vi "ao-amp_test.vi"() -> ()   [LabVIEW 2020]
uses:
  <instrlib>/niDMM/nidmm.llb/niDMM Function.ctl
  <instrlib>/niDMM/nidmm.llb/niDMM Resolution in Digits.ctl
  <instrlib>/niDMM/nidmm.llb/niDMM Configure Measurement Digits.vi
panel:
  in  "Relay 2":refnum<visa-resource-name>="PXI3::9::INSTR"
  in  "Matrix 3":refnum<visa-resource-name>="PXI14::13::INSTR"
  in  "Matrix 2":refnum<visa-resource-name>="PXI14::13::INSTR"
  in  "Resolution in Digits":T1=5.5 items=["3 1/2"=3.5, "4 1/2"=4.5, "5 1/2"=5.5, "6 1/2"=6.5, "7 1/2"=7.5]
  in  "Measurement Type":T2
  out "Signal Out of Range":bool
  in  "Device Name":refnum<k15>="Multimeter"
  in  "Range (Volts)":dbl=10.0 format="%.2p"
  out "Measurement (Volts)":dbl format="%_7p"
  out "error out":errorcluster
  in  "Relay":refnum<visa-resource-name>="PXI3::9::INSTR"
  in  "Matrix":refnum<visa-resource-name>="PXI14::13::INSTR"
  in  "Gain (x1)":u32(ring)=1 items=["x1"=1, "x2"=2, "x5"=3, "x7"=4, "x10"=5, "x14"=6, "x20"=7]
  in  "Channel (CH1)":u32(ring)=1 items=["CH1"=1, "CH2"=2, "CH3"=3, "CH4"=4, "CH5"=5]
  in  "amplifier":refnum<visa-resource-name>="PXI23::10::INSTR" caption="resource name"
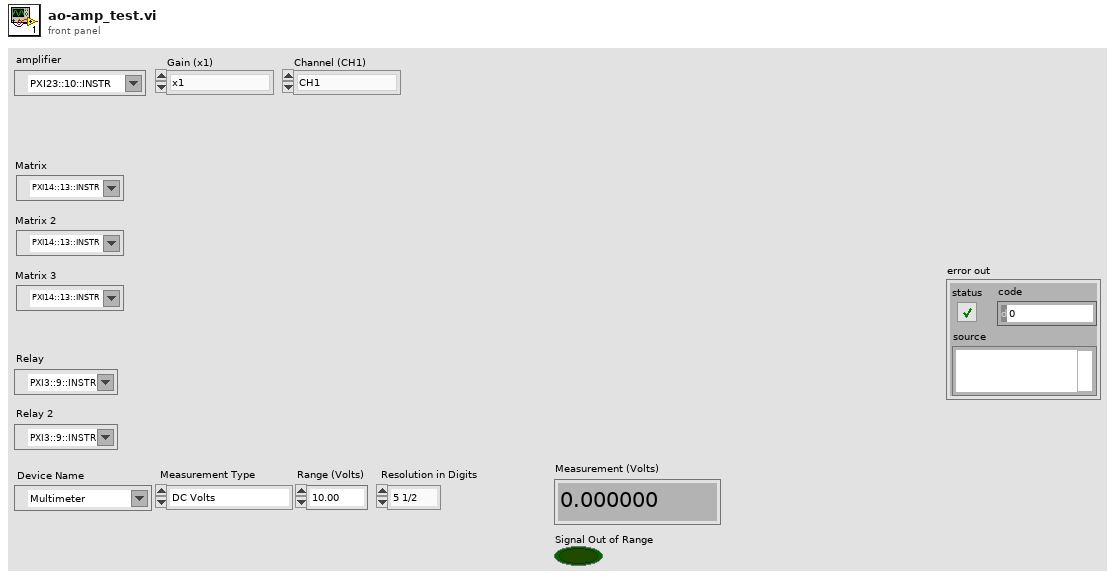
[diagram p1: front panel]
types:
  T1 = typedef "niDMM Resolution in Digits.ctl" = dbl
  T2 = typedef "niDMM Function.ctl" = enum16{"DC Volts", "AC Volts", "DC Current", "AC Current", "2-wire Resistance", "4-wire Resistance", "Diode", "Frequency", "Period", "AC Volts DC Coupled", "Capacitance", "Inductance", "Temperature"}
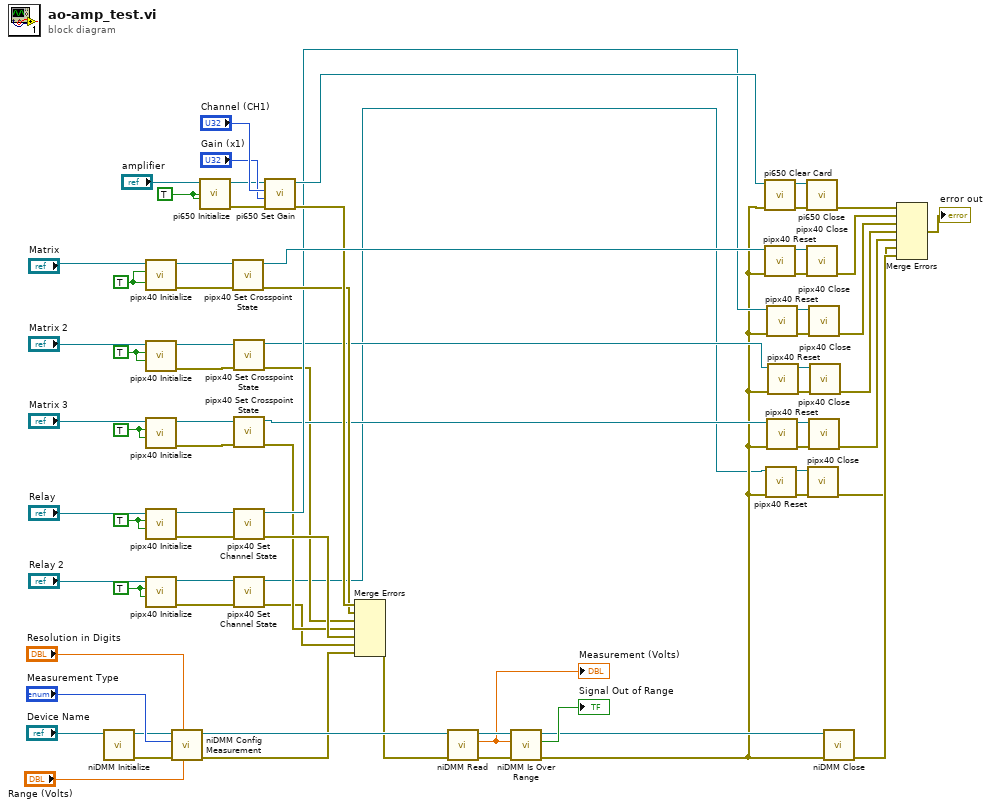
[diagram p0: block diagram]
diagram:
  w14 = TRUE ("id query")
  w25 = TRUE ("id query")
  w26 = TRUE ("id query")
  w50 = TRUE ("id query")
  w63 = TRUE
  w72 = TRUE ("id query (Do Query)")
  n1 = call <instrlib>:"niDMM Initialize.vi"("Instrument Descriptor"="Device Name") -> ("error out"=w33:errorcluster, "instrument handle out"=w32:refnum<k15>)  [unwired: 9 in]
  n2 = call <instrlib>:"pipx40 Initialize.vi"("reset device"=w63, "id query"=w63, "resource name"="Matrix") -> ("error out"=w60:errorcluster, "instrument handle out"=w59:refnum<visa-resource-name>)  [unwired: 7 in]
  n3 = call <instrlib>:"pipx40 Initialize.vi"("reset device"=w26, "id query"=w26, "resource name"="Matrix 2") -> ("error out"=w30:errorcluster, "instrument handle out"=w28:refnum<visa-resource-name>)  [unwired: 7 in]
  n4 = call <instrlib>:"pipx40 Initialize.vi"("reset device"=w25, "id query"=w25, "resource name"="Matrix 3") -> ("error out"=w29:errorcluster, "instrument handle out"=w27:refnum<visa-resource-name>)  [unwired: 7 in]
  n5 = call <instrlib>:"pipx40 Initialize.vi"("reset device"=w50, "id query"=w50, "resource name"="Relay") -> ("error out"=w51:errorcluster, "instrument handle out"=w52:refnum<visa-resource-name>)  [unwired: 7 in]
  n6 = call <instrlib>:"pipx40 Initialize.vi"("reset device"=w14, "id query"=w14, "resource name"="Relay 2") -> ("error out"=w13:errorcluster, "instrument handle out"=w12:refnum<visa-resource-name>)  [unwired: 7 in]
  n7 = call-poly <instrlib>:"niDMM Config Measurement.vi"("Range"="Range (Volts)", "Resolution in Digits"="Resolution in Digits", "error in (no error)"=w33, "Function"="Measurement Type", "instrument handle"=w32) -> ("error out"=w8:errorcluster, "instrument handle out"=w40:refnum<k15>)  [unwired: 5 in]
  n8 = call <instrlib>:"pi650 Initialize.vi"("reset device (Reset Device)"=w72, "id query (Do Query)"=w72, "resource name"="amplifier") -> ("error out"=w66:errorcluster, "instrument handle out"=w67:refnum<visa-resource-name>)  [unwired: 7 in]
  n9 = call <instrlib>:"pipx40 Set Crosspoint State.vi"("error in (no error)"=w60, "instrument handle"=w59) -> ("error out"=w56:errorcluster, "instrument handle out"=w58:refnum<visa-resource-name>)  [unwired: 8 in]
  n10 = call <instrlib>:"pipx40 Set Crosspoint State.vi"("error in (no error)"=w30, "instrument handle"=w28) -> ("error out"=w10:errorcluster, "instrument handle out"=w16:refnum<visa-resource-name>)  [unwired: 8 in]
  n11 = call <instrlib>:"pipx40 Set Crosspoint State.vi"("error in (no error)"=w29, "instrument handle"=w27) -> ("error out"=w9:errorcluster, "instrument handle out"=w15:refnum<visa-resource-name>)  [unwired: 8 in]
  n12 = call <instrlib>:"pipx40 Set Channel State.vi"("error in (no error)"=w51, "instrument handle"=w52) -> ("error out"=w49:errorcluster, "instrument handle out"=w45:refnum<visa-resource-name>)  [unwired: 8 in]
  n13 = call <instrlib>:"pipx40 Set Channel State.vi"("error in (no error)"=w13, "instrument handle"=w12) -> ("error out"=w7:errorcluster, "instrument handle out"=w1:refnum<visa-resource-name>)  [unwired: 8 in]
  n14 = call <instrlib>:"pi650 Set Gain.vi"("error in (no error)"=w66, "Gain (x1)"="Gain (x1)", "Channel (CH1)"="Channel (CH1)", "instrument handle"=w67) -> ("error out"=w57:errorcluster, "instrument handle out"=w65:refnum<visa-resource-name>)  [unwired: 6 in]
  n15 = Merge Errors(w57, w56, w10, w9, w49, w7, w8) -> (w31:errorcluster)
  n16 = call <instrlib>:"niDMM Read.vi"("error in (no error)"=w31, "instrument handle"=w40) -> ("error out"=w39:errorcluster, "Measurement"=w37:dbl, "instrument handle out"=w38:refnum<k15>)  [unwired: 7 in]
  "Measurement (Volts)" <- w37
  n17 = call <instrlib>:"niDMM Is Over Range.vi"("error in (no error)"=w39, "Measurement"=w37, "instrument handle"=w38) -> ("error out"=w5:errorcluster, "Over Range?"=→"Signal Out of Range":bool, "instrument handle out"=w41:refnum<k15>)  [unwired: 6 in]
  n18 = call <instrlib>:"pi650 Clear Card.vi"("error in (no error)"=w5, "instrument handle"=w65) -> ("error out"=w71:errorcluster, "instrument handle out"=w70:refnum<visa-resource-name>)  [unwired: 8 in]
  n19 = call <instrlib>:"pipx40 Reset.vi"("error in (no error)"=w5, "instrument handle"=w58) -> ("error out"=w61:errorcluster, "instrument handle out"=w62:refnum<visa-resource-name>)  [unwired: 8 in]
  n20 = call <instrlib>:"pipx40 Reset.vi"("error in (no error)"=w5, "instrument handle"=w1) -> ("error out"=w6:errorcluster, "instrument handle out"=w2:refnum<visa-resource-name>)  [unwired: 8 in]
  n21 = call <instrlib>:"pipx40 Reset.vi"("error in (no error)"=w5, "instrument handle"=w45) -> ("error out"=w48:errorcluster, "instrument handle out"=w46:refnum<visa-resource-name>)  [unwired: 8 in]
  n22 = call <instrlib>:"pipx40 Reset.vi"("error in (no error)"=w5, "instrument handle"=w15) -> ("error out"=w20:errorcluster, "instrument handle out"=w19:refnum<visa-resource-name>)  [unwired: 8 in]
  n23 = call <instrlib>:"pipx40 Reset.vi"("error in (no error)"=w5, "instrument handle"=w16) -> ("error out"=w21:errorcluster, "instrument handle out"=w22:refnum<visa-resource-name>)  [unwired: 8 in]
  n24 = call <instrlib>:"pi650 Close.vi"("error in (no error)"=w71, "instrument handle"=w70) -> ("error out"=w55:errorcluster)  [unwired: 9 in]
  n25 = call <instrlib>:"pipx40 Close.vi"("error in (no error)"=w61, "instrument handle"=w62) -> ("error out"=w54:errorcluster)  [unwired: 9 in]
  n26 = call <instrlib>:"pipx40 Close.vi"("error in (no error)"=w6, "instrument handle"=w2) -> ("error out"=w3:errorcluster)  [unwired: 9 in]
  n27 = call <instrlib>:"pipx40 Close.vi"("error in (no error)"=w48, "instrument handle"=w46) -> ("error out"=w47:errorcluster)  [unwired: 9 in]
  n28 = call <instrlib>:"pipx40 Close.vi"("error in (no error)"=w20, "instrument handle"=w19) -> ("error out"=w17:errorcluster)  [unwired: 9 in]
  n29 = call <instrlib>:"pipx40 Close.vi"("error in (no error)"=w21, "instrument handle"=w22) -> ("error out"=w18:errorcluster)  [unwired: 9 in]
  n30 = call <instrlib>:"niDMM Close.vi"("error in (no error)"=w5, "instrument handle"=w41) -> ("error out"=w4:errorcluster)  [unwired: 9 in]
  n31 = Merge Errors(w55, w54, w47, w18, w17, w3, w4) -> (→"error out":errorcluster)
